vi "usrp_driver.vi"() -> ()   [LabVIEW 2021]
doc: "This template is for the Simple NI-USRP Streaming design, a design that shows the basics of streaming data to and from an NI USRP-294x/295x device. Refer to the block diagram for more information about how to use this template."
uses:
  <instrlib>/niUSRP/niUSRP Fetch Rx Data (I16).vi
panel:
  out "total record time(ms)":u32
  in  "active antenna":string="RX1"
  out "coerced IQ rate":dbl=100000.0 format="%#_6p"
  out "buffer size(s)":i32 format="%.0p"
  in  "Device Name":refnum<k15>="192.168.10.2"
  out "write rate (KSPS)":dbl
  out "# elements in queue":i32
  out "write tdms loop time":u32
  in  "frequency":dbl=2000000000.0 format="%#_6p"
  in  "sample rate":i32=50000000 format="%.0p"
  out "get data loop time":u32 format="%.0p"
  out "error tdms_loop":errorcluster
  out "acquiring":bool caption="Streaming"
  in  "rx.stop":bool
  # "Overview: Demonstrates the use of the Advanced TDMS and simple streamer functions to write Rx data to a *.tdms file.\nInstructions:\nThis Vi must use Administrator privliges in order to write the data.\nthe USRP sohld be connected via MIXe to the computer (or other direct connection)\nset the params \nRun this VI.\ndeu to the way the memory work after some time it can occer that the saveing rate will decrise."
  # "Rx Streaming"
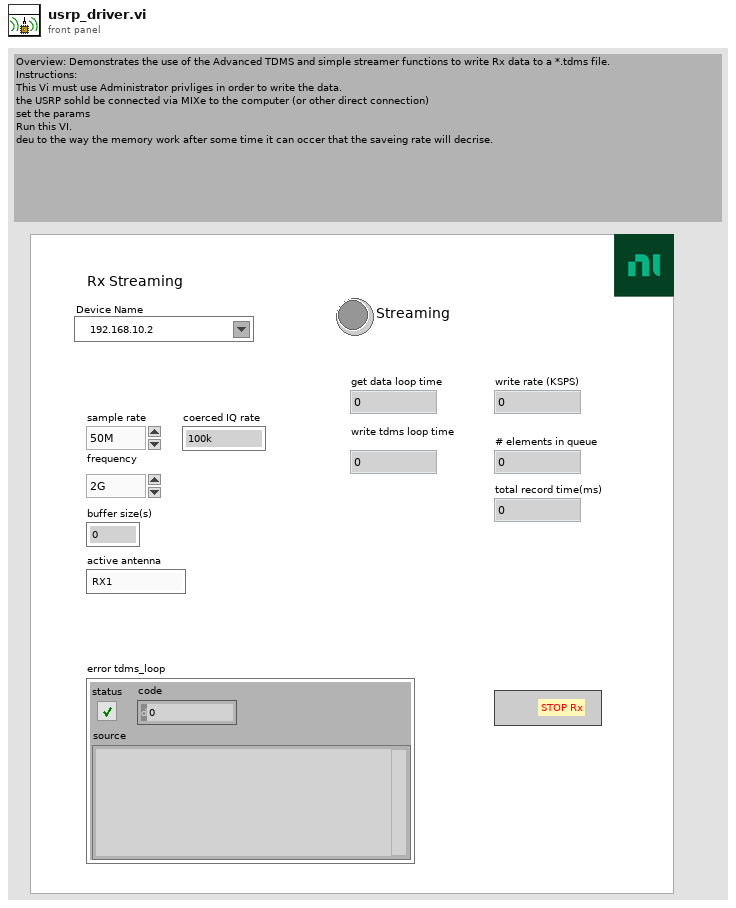
[diagram p1: front panel]
types:
  T1 = enum16{"open", "open or create", "create or replace", "create", "open (read-only)"}
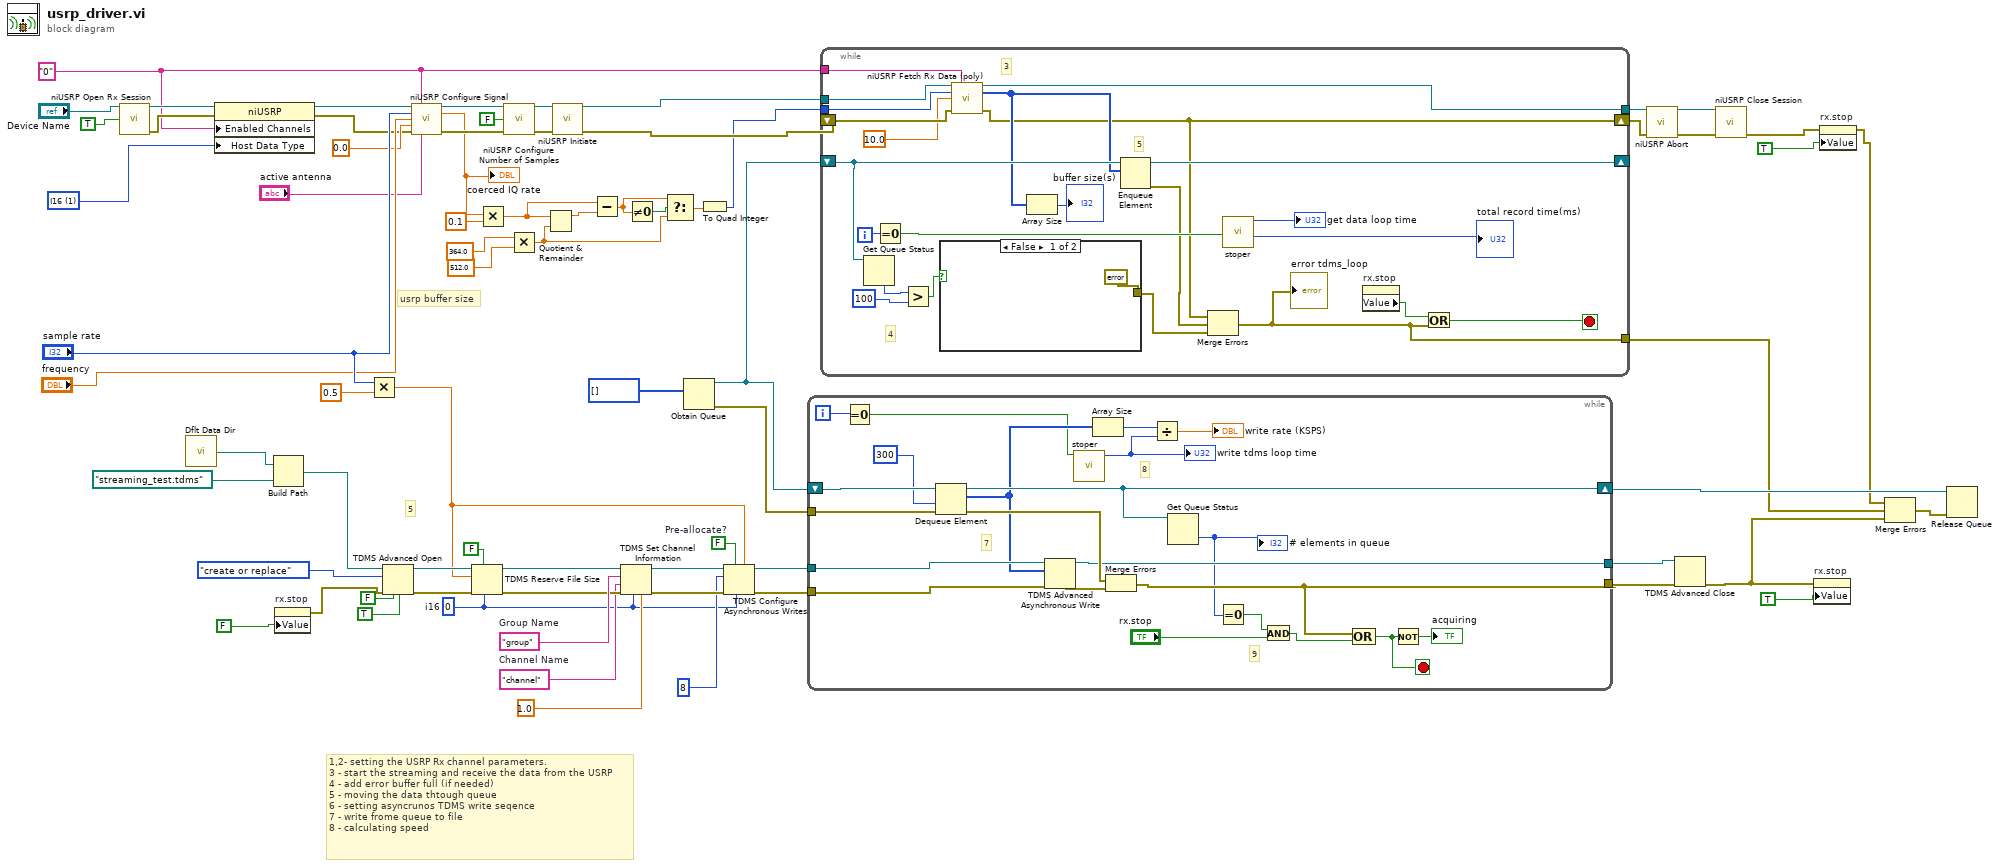
[diagram p0: block diagram]
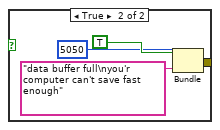
[diagram p2: hidden frame]
diagram:
  w16 = "0" ("Configuration:Enabled Channels")
  w40 = 1 items=["CDB", "I16"] ("Configuration:Advanced:Host Data Type")
  w62 = FALSE  # Pre-allocate?
  w48 = i16 0  # i16
  w72 = "group"  # Group Name
  w50 = "channel"  # Channel Name
  # "usrp buffer size"
  # "1,2- setting the USRP Rx channel parameters.\n3 - start the streaming and receive the data from the USRP\n4 - add error buffer full (if needed)\n5 - moving the data thtough queue   \n6 - setting asyncrunos TDMS write seqence\n7 - write frome queue to file\n8 - calculating speed"
  # "5"
  n1 = call <instrlib>:"niUSRP Open Rx Session.vi"("device names"="Device Name", "reset"=TRUE) -> ("session handle out"=w32:refnum<k15>, "error out"=w33:errorcluster)  [unwired: 12 in]
  n2 = call <vilib>:"Dflt Data Dir.vi"() -> ("App:Default Data Directory"=w36:path)
  n3 = property class="niUSRP"(reference=w32, error in=w33, "Enabled Channels"=w16, "Host Data Type"=w40) -> (reference out=w29:refnum<k15>, error out=w25:errorcluster)
  n4 = Build Path(base path=w36, name or relative path=path "streaming_test.tdms") -> (appended path=w35:path)
  n5 = property on="rx.stop" class="Bool (strict)"("Value"=FALSE) -> (error out=w44:errorcluster)  [unwired: 2 in, 1 out]
  n6 = Multiply(x="sample rate", y=0.5) -> (x*y=w51:dbl)
  n7 = TDMS Advanced Open(4:TRUE ("enable asynchronous? (T)"), 6:FALSE ("disable buffering? (T)"), 8:w44, 10:T1."create or replace" ("operation (0:open)"), 11:w35) -> (0:w68:errorcluster, 3:w69:refnum<k34>)  [unwired: 1 out]
  n8 = call <instrlib>:"niUSRP Configure Signal.vi"("session handle"=w29, "channel list"=w16, "IQ rate"="sample rate", "carrier frequency"="frequency", "gain"=0.0, "error in (no error)"=w25, "active antenna"="active antenna") -> ("session handle out"=w23:refnum<k15>, "coerced IQ rate"=w14:dbl, "error out"=w24:errorcluster)  [unwired: 4 in, 2 out]
  "coerced IQ rate" <- w14
  n9 = TDMS Reserve File Size(6:w48, 7:FALSE ("append? (T)"), 8:w68, 10:w51, 11:w69) -> (0:w66:errorcluster, 3:w67:refnum<k34>)
  n10 = Multiply(x=w14, y=0.1) -> (x*y=w12:dbl)
  n11 = call <instrlib>:"niUSRP Configure Number of Samples.vi"("session handle"=w23, "number of samples is finite"=FALSE, "error in (no error)"=w24) -> ("session handle out"=w20:refnum<k15>, "error out"=w21:errorcluster)  [unwired: 11 in]
  n12 = Multiply(x=364.0 ("y"), y=512.0) -> (x*y=w4:dbl)
  n13 = Quotient & Remainder(x=w12, y=w4) -> (x-y*floor(x/y)=w11:dbl)  [unwired: 1 out]
  n14 = call <instrlib>:"niUSRP Initiate.vi"("session handle"=w20, "error in (no error)"=w21) -> ("session handle out"=w19:refnum<k15>, "error out"=w22:errorcluster)  [unwired: 12 in]
  n15 = Subtract(x=w12, y=w11) -> (x-y=w5:dbl)
  n16 = TDMS Set Channel Information(4:1.0 ("y"), 6:w48, 8:w66, 9:w50, 10:w72, 11:w67) -> (0:w64:errorcluster, 3:w63:refnum<k34>)  [unwired: 1 in]
  n17 = Not Equal To 0?(x=w5) -> (x != 0?=w6:bool)
  n18 = Select(t=w5, s=w6, f=w4) -> (s? t:f=w7:dbl)
  n19 = Obtain Queue(element data type=i16[] [] ("waveform data")) -> (queue out=w57:refnum<queue>, error out=w56:errorcluster)  [unwired: 4 in, 1 out]
  n20 = To Quad Integer(1:w7) -> (0:w10:i64)
  n21 = TDMS Configure Asynchronous Writes(5:w51, 6:w48, 7:w62, 8:w64, 10:u32 8 ("max asynchronous writes (4)"), 11:w63) -> (0:w52:errorcluster, 3:w59:refnum<k34>)  [unwired: 1 in]
  n22 = while {
    tunnel: w59 -> [w92]
    shift-right: [w83] -> w53
    shift-left: w57 -> [w91]
    tunnel: w56 -> [w84]
    tunnel: [w89] -> w43
    tunnel: [w88] -> w54
    tunnel: w52 -> [w86]
    i -> [w74]
    stop <- w87 stop-if-true
    # "9"
    # "8"
    # "7"
    n23 = Equal To 0?(x=w74) -> (x = 0?=w73:bool)
    n24 = Dequeue Element(queue=w91, timeout in ms (-1)=300, error in (no error)=w84) -> (queue out=w83:refnum<queue>, element=w75:i16[], error out=w90:errorcluster)  [unwired: 1 out]
    n25 = TDMS Advanced Asynchronous Write(8:w86, 10:w75, 11:w92) -> (0:w93:errorcluster, 3:w88:refnum<k34>)
    n26 = call "stoper.vi"("start"=w73) -> ("loop"=w76:u32)  [unwired: 9 in, 1 out]
    "write tdms loop time" <- w76
    n27 = Array Size(array=w75) -> (size(s)=w78:i32)
    n28 = Merge Errors(w90, w93) -> (w89:errorcluster)
    n29 = Divide(x=w78, y=w76) -> (x/y=→"write rate (KSPS)":dbl)
    n30 = Get Queue Status(queue=w83) -> (# elements in queue=w82:i32)  [unwired: 2 in, 7 out]
    "# elements in queue" <- w82
    n31 = Equal To 0?(x=w82) -> (x = 0?=w81:bool)
    n32 = And(x=w81, y="rx.stop") -> (x .and. y?=w80:bool)
    n33 = Compound Arithmetic op=OR(w89, w80) -> (w87:bool)
    n34 = Not(x=w87) -> (.not. x?=→"acquiring":bool)
  }
  n35 = while {
    shift-right: [w113] -> _
    shift-left: w57 -> [w109]
    tunnel: [w110] -> w41
    tunnel: w19 -> [w101]
    tunnel: w16 -> [w102]
    tunnel: w10 -> [w100]
    shift-right: [w97] -> w17
    shift-left: w22 -> [w103]
    tunnel: [w99] -> w18
    i -> [w117]
    stop <- w115 stop-if-true
    # "5"
    # "4"
    # "3"
    # "Acquire and Fetch a waveform"
    n36 = Get Queue Status(queue=w109) -> (# elements in queue=w108:i32)  [unwired: 2 in, 7 out]
    n37 = Equal To 0?(x=w117) -> (x = 0?=w116:bool)
    n38 = Greater?(x=w108, y=100) -> (0:w106:bool)
    n39 = case shown="False" w106 {
      tunnel: [errorcluster {"status"=FALSE, "code"=0, "source"=""} ("error out") w122] -> w105
      frame False {
      }
      frame True {
        n40 = Bundle("status"=TRUE, "code"=5050, "source"="data buffer full\nyou'r computer can't save fast enough") -> (w122:errorcluster)  [unwired: 1 in]
      }
    }
    n41 = call-poly <instrlib>:"niUSRP Fetch Rx Data (poly).vi"("session handle"=w101, "channel list"=w102, "number of samples"=w100, "timeout"=10.0, "error in (no error)"=w103) -> ("session handle out"=w99:refnum<k15>, "data"=w98:i16[], "error out"=w97:errorcluster)  [unwired: 7 in, 1 out]
    n42 = Array Size(array=w98) -> (size(s)=→"buffer size(s)":i32)
    n43 = Enqueue Element(queue=w109, element=w98) -> (queue out=w113:refnum<queue>, error out=w111:errorcluster)  [unwired: 2 in, 1 out]
    n44 = Merge Errors(w97, w111, w105) -> (w110:errorcluster)
    "error tdms_loop" <- w110
    n45 = call "stoper.vi"("start"=w116) -> ("frome start"=→"total record time(ms)":u32, "loop"=→"get data loop time":u32)  [unwired: 9 in]
    n46 = property on="rx.stop" class="Bool (strict)"() -> ("Value"=w114:bool)  [unwired: 2 in, 2 out]
    n47 = Or(x=w114, y=w110) -> (x .or. y?=w115:bool)
  }
  n48 = call <instrlib>:"niUSRP Abort.vi"("session handle"=w18, "error in (no error)"=w17) -> ("session handle out"=w38:refnum<k15>, "error out"=w39:errorcluster)  [unwired: 12 in]
  n49 = TDMS Advanced Close(8:w43, 11:w54) -> (0:w42:errorcluster)  [unwired: 2 in, 1 out]
  n50 = call <instrlib>:"niUSRP Close Session.vi"("session handle"=w38, "error in (no error)"=w39) -> ("error out"=w3:errorcluster)  [unwired: 13 in]
  n51 = property on="rx.stop" class="Bool (strict)"(error in=w42, "Value"=TRUE) -> ()  [unwired: 1 in, 2 out]
  n52 = property on="rx.stop" class="Bool (strict)"(error in=w3, "Value"=TRUE) -> (error out=w1:errorcluster)  [unwired: 1 in, 1 out]
  n53 = Merge Errors(w1, w41, w42) -> (w45:errorcluster)
  n54 = Release Queue(queue=w53, error in (no error)=w45) -> ()  [unwired: 1 in, 3 out]
